vi "Analog Input.vi"() -> ()   [LabVIEW 2022 SP3]
uses:
  <vilib>/DAQmx/read.llb/DAQmx Read (Analog 2D DBL NChan NSamp).vi
  <vilib>/DAQmx/create/channels.llb/DAQmx Create Channel (AI-Voltage-Basic).vi
  <vilib>/DAQmx/miscellaneous.llb/DAQmx Fill In Error Info.vi
panel:
  out "data":dbl[][](array[numeric]) format="%0.2f"
  in  "stop":bool
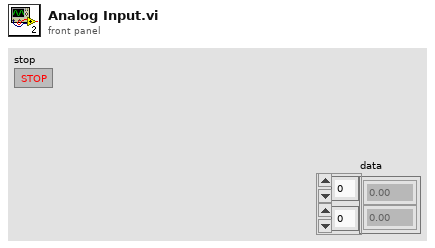
[diagram p1: front panel]
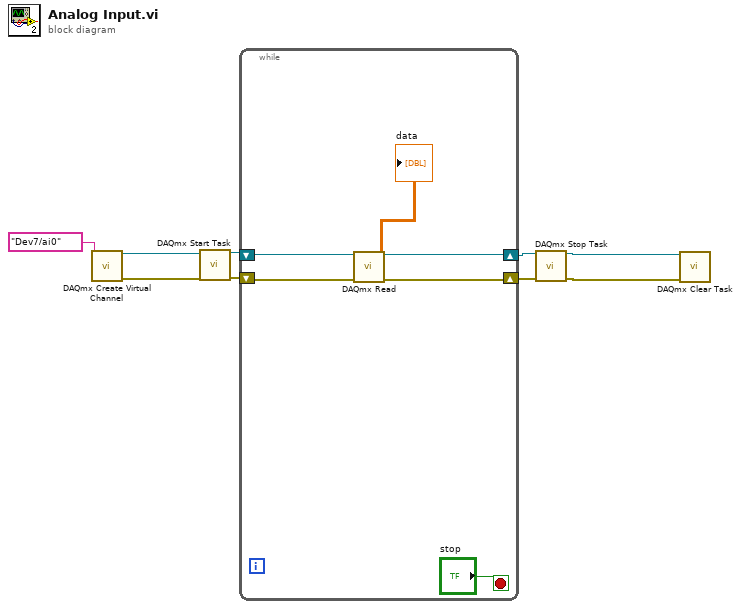
[diagram p0: block diagram]
diagram:
  n1 = call-poly <vilib>:"DAQmx Create Virtual Channel.vi"("physical channels"=tag "Dev7/ai0") -> ("task out"=w9:refnum<k21>, "error out"=w5:errorcluster)  [unwired: 13 in]
  n2 = call <vilib>:"DAQmx Start Task.vi"("task/channels in"=w9, "error in"=w5) -> ("task out"=w8:refnum<k21>, "error out"=w4:errorcluster)  [unwired: 12 in]
  n3 = while {
    shift-right: [w12] -> w7
    shift-left: w8 -> [w14]
    shift-right: [w11] -> w3
    shift-left: w4 -> [w13]
    stop <- "stop" stop-if-true
    n4 = call-poly <vilib>:"DAQmx Read.vi"("task/channels in"=w14, "error in"=w13) -> ("task out"=w12:refnum<k21>, "data"=→"data":dbl[][], "error out"=w11:errorcluster)  [unwired: 11 in]
  }
  n5 = call <vilib>:"DAQmx Stop Task.vi"("task/channels in"=w7, "error in"=w3) -> ("task out"=w6:refnum<k21>, "error out"=w2:errorcluster)  [unwired: 12 in]
  n6 = call <vilib>:"DAQmx Clear Task.vi"("task in"=w6, "error in"=w2) -> ()  [unwired: 13 in, 1 out]
